vi "SDCP BTR Parameter FGV.vi"(4 "error in (no error)":errorcluster, 5 "Command":enum16{"Load", "Read", "Write"}(ring), 6 "BTR Parameter File Path":path, 7 "BTRP in":T1[](array[typedef])) -> (0 "error out":errorcluster, 3 "BTRP out":T1[](array[typedef]))   [LabVIEW 2020]
uses:
  Typedefs/SDCP BTR Parameter cluster.ctl
  Typedefs/SDCP BTR Parameter data type.ctl
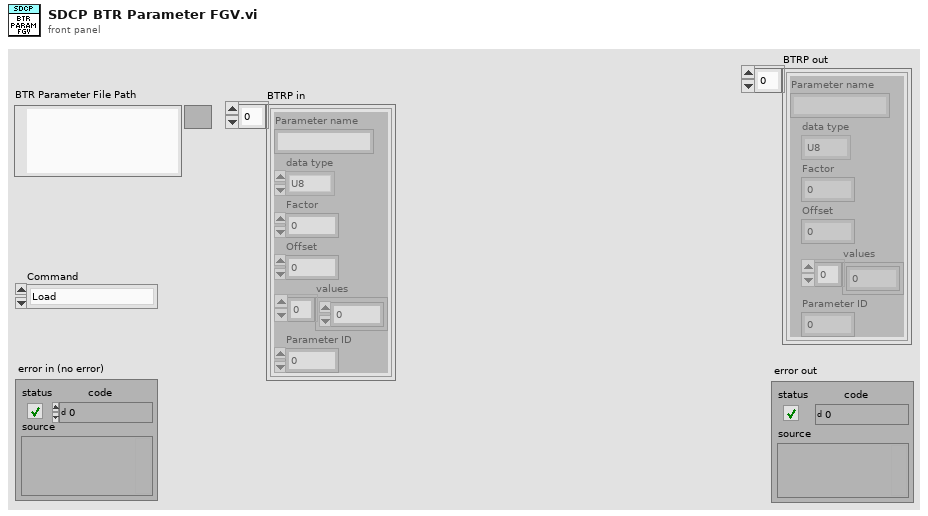
[diagram p1: front panel]
types:
  T1 = typedef "SDCP BTR Parameter cluster.ctl" = cluster{"Parameter name":string, "data type":T2, "Factor":dbl, "Offset":dbl, "values":dbl[], "Parameter ID":i32}
  T2 = typedef "SDCP BTR Parameter data type.ctl" = enum16{"U8", "I8", "U16", "I16", "U32", "I32", "F32"}
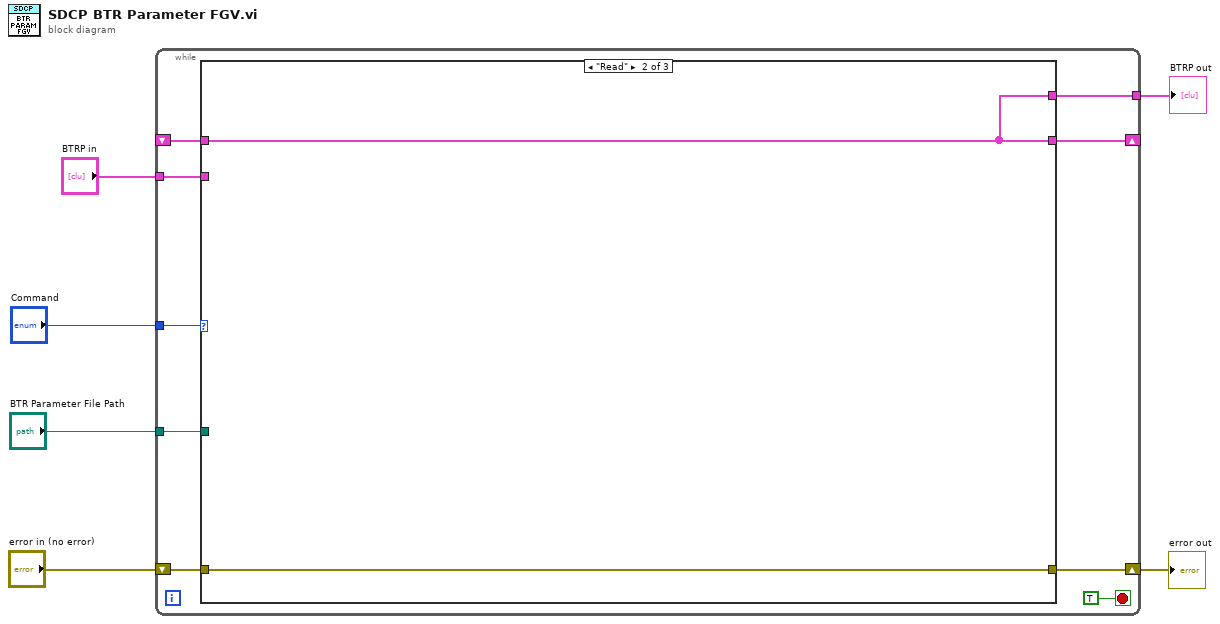
[diagram p0: block diagram]
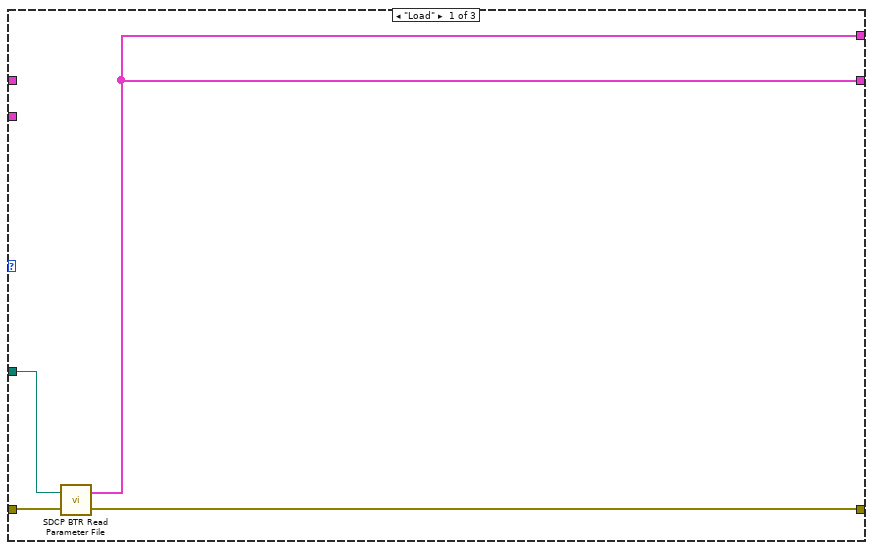
[diagram p2: hidden frame]
diagram:
  n1 = while {
    shift-right: [w12] -> w5
    shift-left: "error in (no error)" -> [w14]
    tunnel: "Command" -> [w13]
    tunnel: "BTR Parameter File Path" -> [w11]
    shift-right: [w10] -> _
    shift-left: _ -> [w9]
    tunnel: [w8] -> w2
    tunnel: "BTRP in" -> [w7]
    stop <- TRUE stop-if-true
    n2 = case shown="\"Read\"" w13 {
      tunnel: w14 -> [w19 w20 w22]
      tunnel: [w17 w20 w22] -> w12
      tunnel: w11 -> [w18 _ _]
      tunnel: [w16 w21 w23] -> w10
      tunnel: w9 -> [_ w21 _]
      tunnel: [w16 w21 w23] -> w8
      tunnel: w7 -> [_ _ w23]
      frame "Load" {
        n3 = call "SDCP BTR Read Parameter File.vi"("error in (no error)"=w19, "BTP File Path"=w18) -> ("error out"=w17:errorcluster, "BTR parameters"=w16:T1[])
      }
      frame "Read" {
      }
      frame "Write" {
      }
    }
  }
  "error out" <- w5
  "BTRP out" <- w2
